vi "Read Test Cases.vi"(11 "Test Suite In":refnum<class "LUnit Test Suite.lvclass">) -> (2 "Test Cases":refnum<class "LUnit Test Case.lvclass">[](array[class]), 3 "Test Suite Out":refnum<class "LUnit Test Suite.lvclass">)   [LabVIEW 2020, in "LUnit Test Suite.lvclass"]
doc: "Get next test case to execute."
uses:
  LUnit Test Suite.lvclass
  Test Case/LUnit Test Case.lvclass
  LUnit Test Suite.lvclass/LUnit Test Suite.ctl
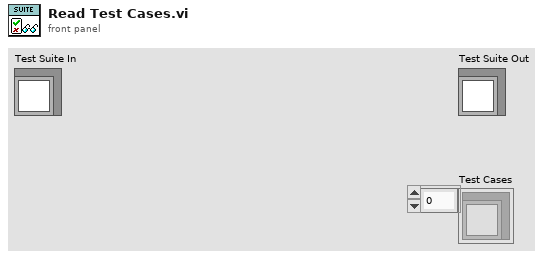
[diagram p1: front panel]
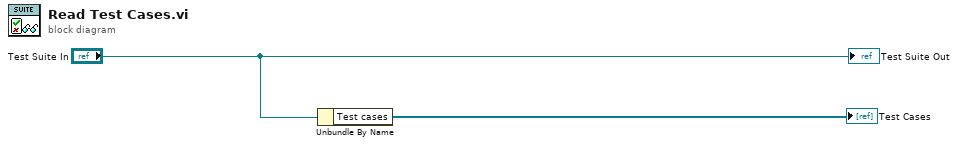
[diagram p0: block diagram]
diagram:
  n1 = Unbundle By Name("Test Suite In") -> ("Test cases"=→"Test Cases":refnum<class "LUnit Test Case.lvclass">[])
  "Test Suite Out" <- "Test Suite In"
